vi "hex_tests.vi"() -> ()   [LabVIEW 2018]
panel:
  out "x > y?":bool
  out "concatenated string 3":string
  out "floor(x/y) 5":u32
  out "x-y*floor(x/y) 5":u32
  out "floor(x/y) 3":u32
  out "x-y*floor(x/y) 3":u32=2
  out "x-y*floor(x/y) 4":u32=12
  out "floor(x/y) 4":u32=18
  out "appended array 2":u32[](array[numeric])=[18, 12]
  out "string 3":string
  in  "y 2":u32=300
  in  "y":u32=300
  out "string 2":string
  out "appended array":u32[](array[numeric])=[1, 200]
  out "x+y":u32=200
  out "floor(x/y) 2":u32=1
  out "unsigned byte array":u8[](array[numeric])=[18, 12]
  out "string":string
  out "floor(x/y)":u32=18
  out "x-y*floor(x/y) 2":u32=2
  out "hex integer string":string="C"
  out "x-y*floor(x/y)":u32=12
  out "value":u32
  out "number":u32
  in  "hex":string="ý"
  out "offset past number 2":i32=1
  out "concatenated string":string
  out "number 3":u32=10
  out "decimal integer string":string="15"
  out "hex integer string 3":string="FFFFFFF1"
  out "hex integer string 2":string="F"
  out "offset past number":i32=1
  out "number 2":u32=9
  # "hex display makes out of 9 => 39"
  # "C"
  # "300 / 16 = 18,75 // 0,75 * 16 = 12"
  # "18 / 16 = 1,125 // 0,125 * 16 = 2"
  # "300 = 12C"
  # "4095 => FF0F wobei FF von unten"
  # "4096  => 0000 wobei unten überlauf bei IQ auf 16"
  # "4097 => 0001"
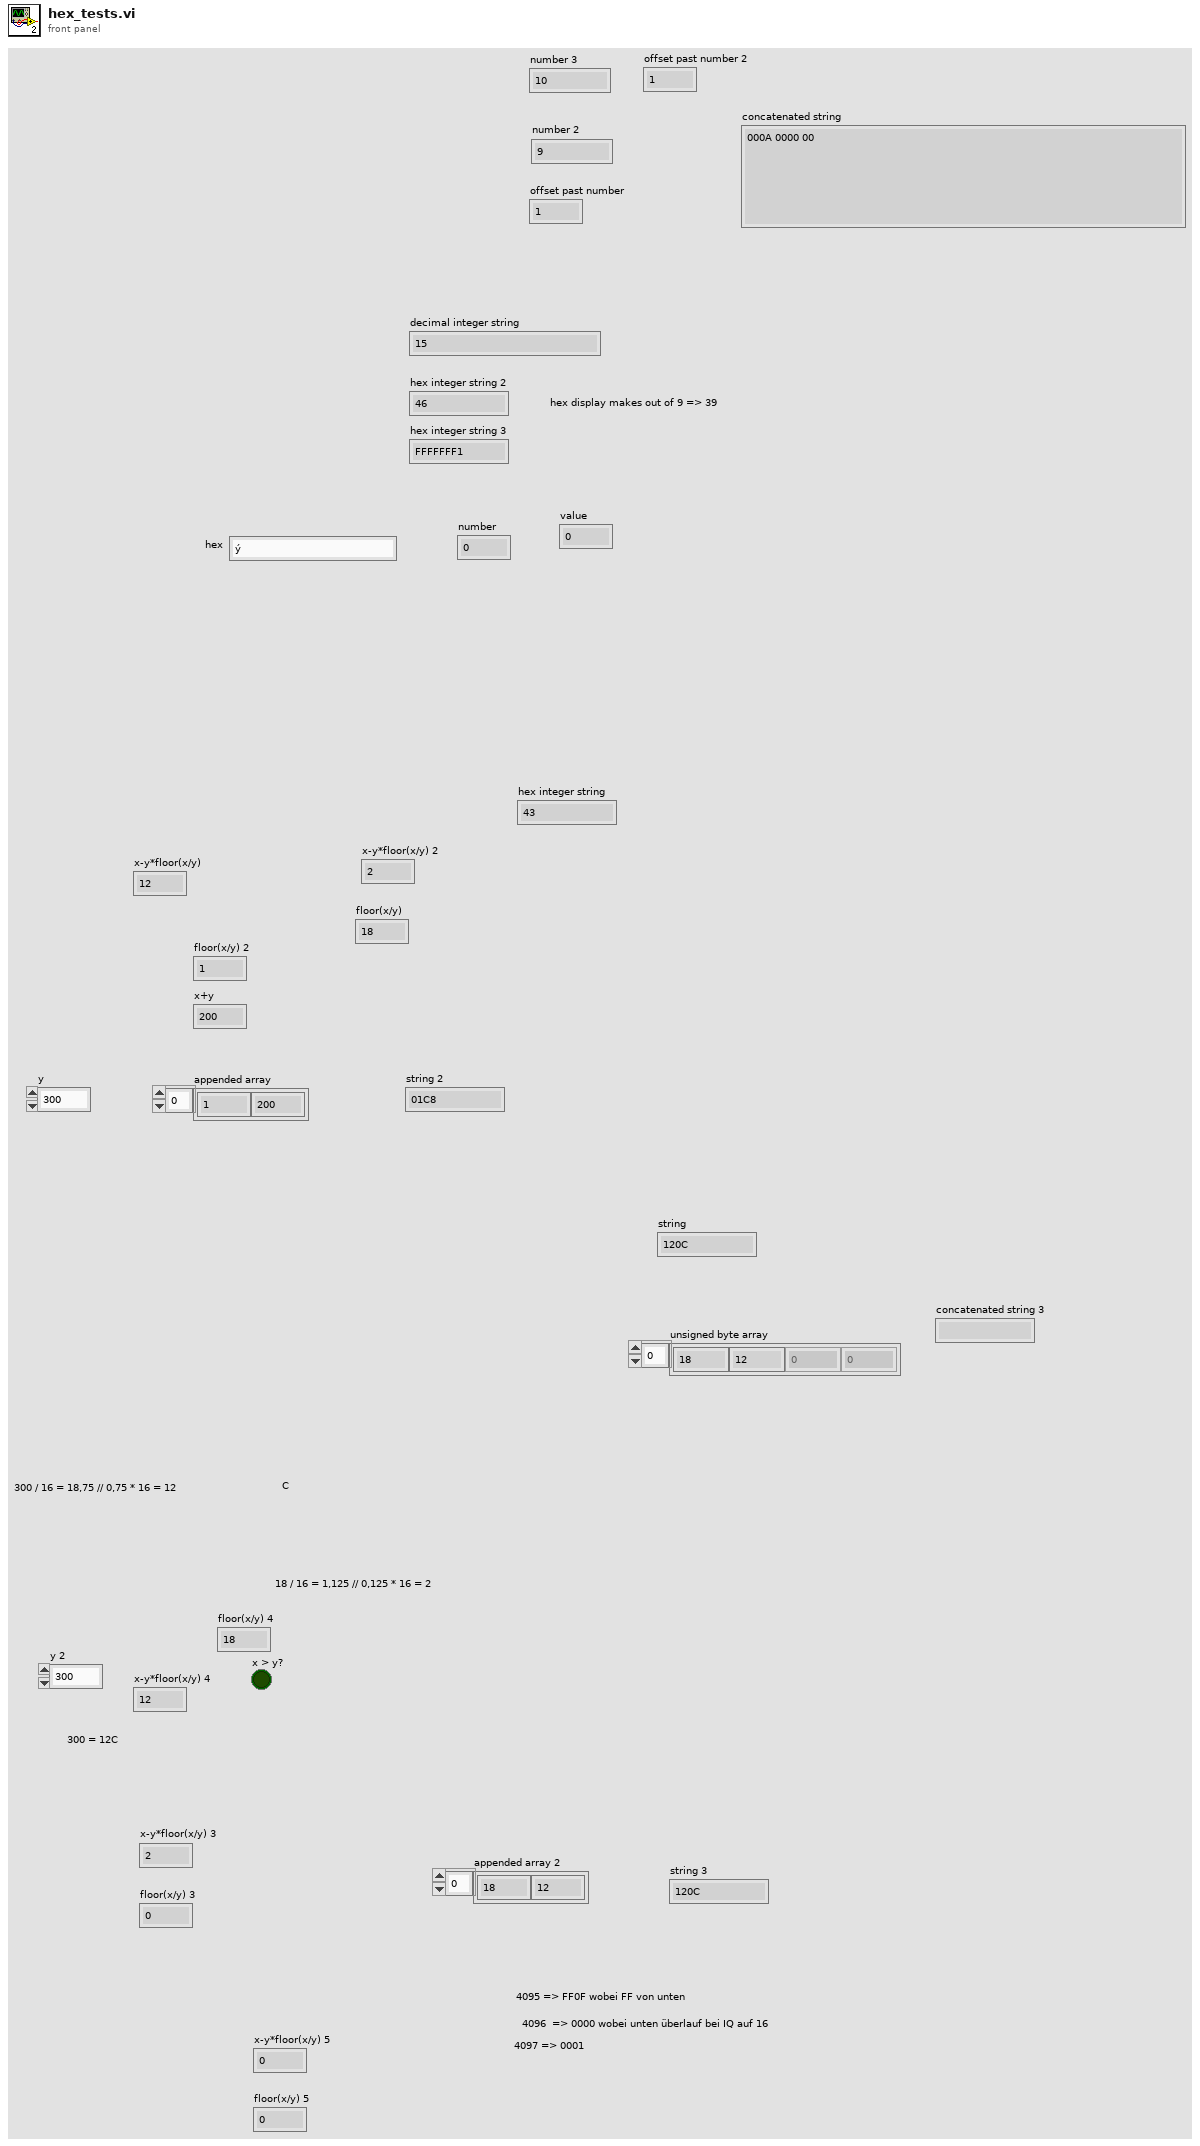
[diagram p1: front panel]
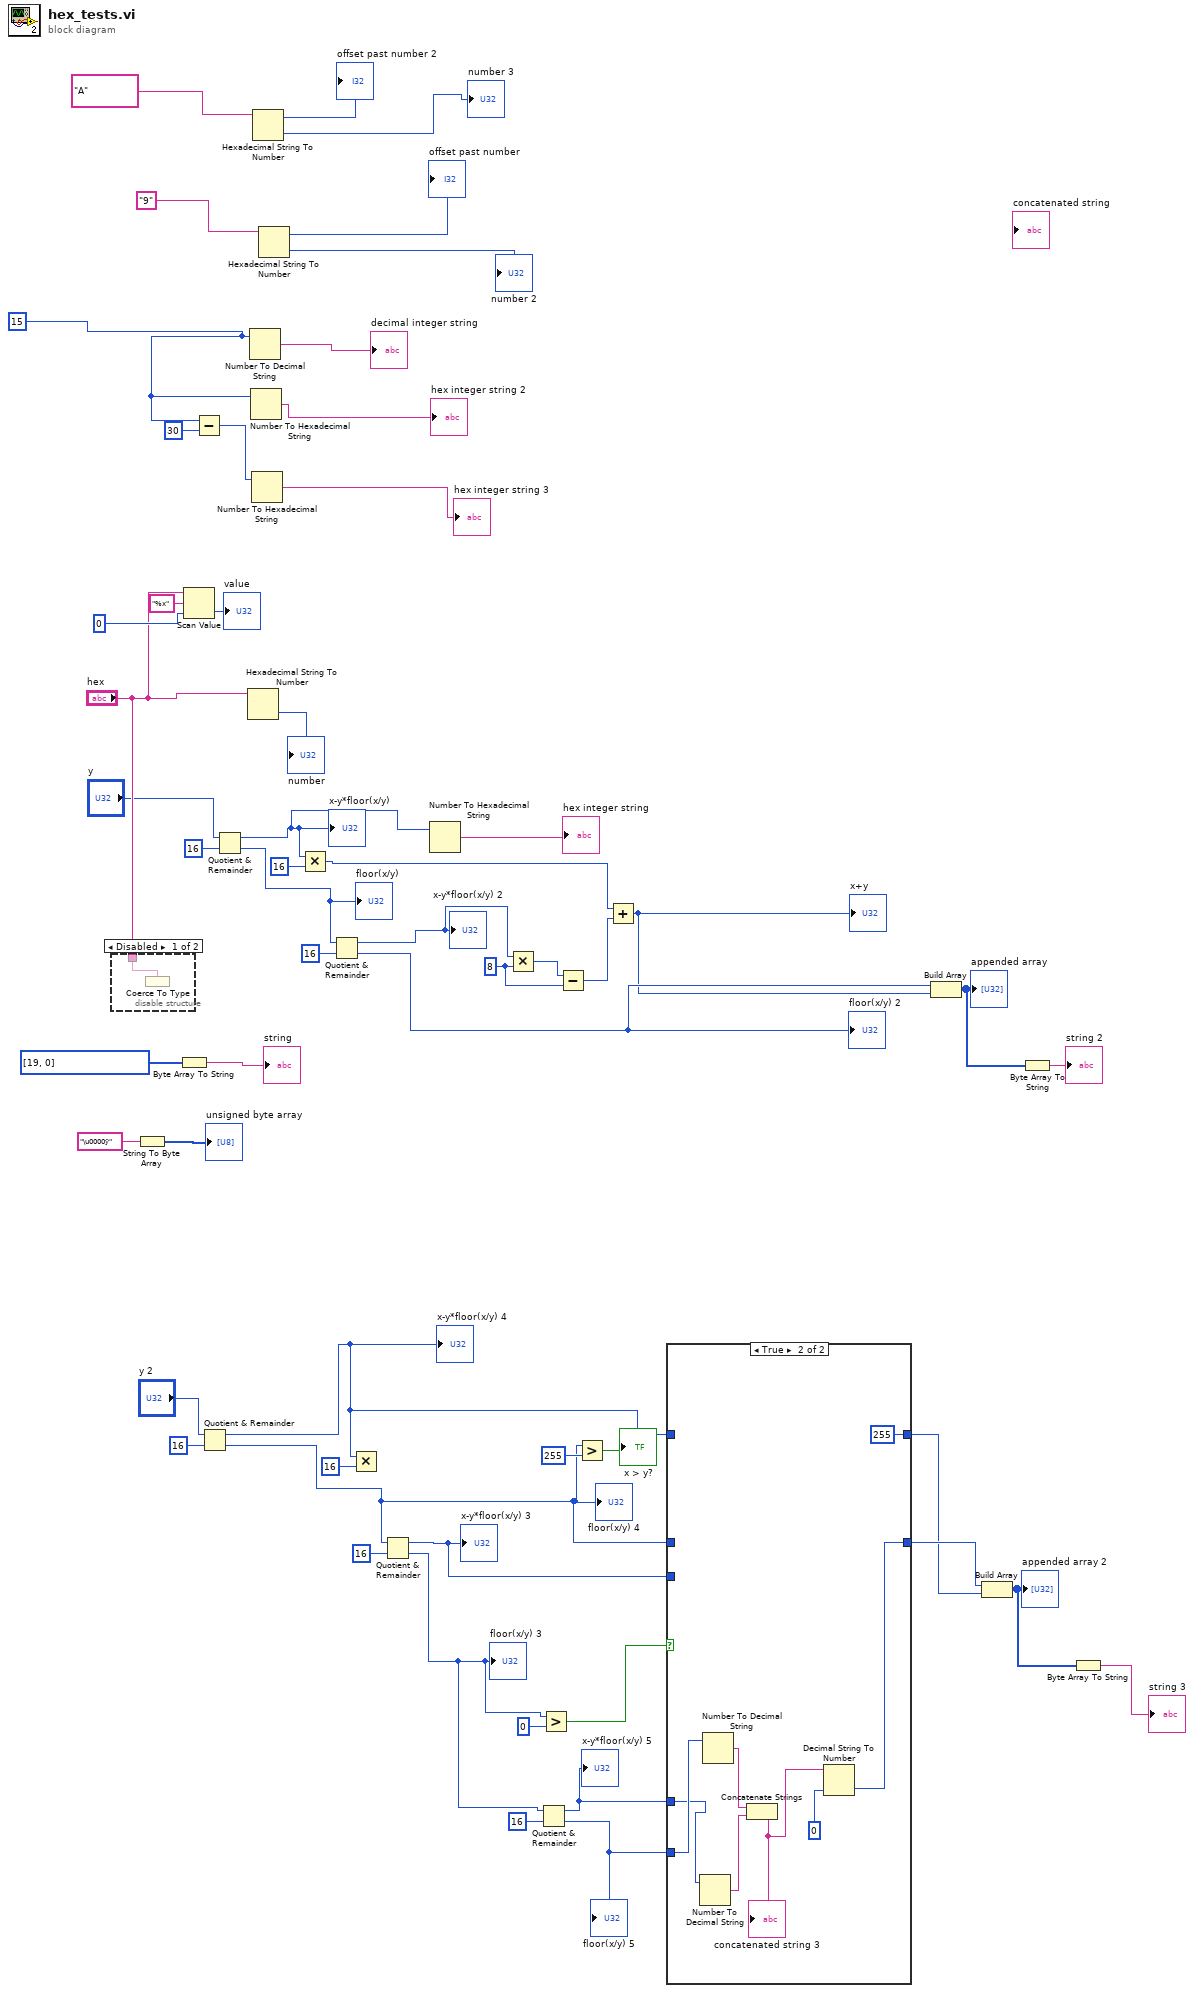
[diagram p0: block diagram]
diagram:
  w20 = u32 8 ("y")
  w45 = u32 15 ("number")
  n1 = disable-structure shown="Disabled" {
    disable-tunnel: "hex" -> [w57 _]
    frame Disabled {
      n2 = Coerce To Type(1:w57) -> ()  [unwired: 1 in, 1 out]
    }
    frame Enabled {
    }
  }
  n3 = String To Byte Array(string="\u0000ÿ") -> (unsigned byte array=→"unsigned byte array":u8[])
  n4 = Byte Array To String(unsigned byte array=u8[] [19, 0]) -> (string=→"string":string)
  n5 = Scan Value(string="hex", format string="%x", default (0 dbl)=u32 0 ("default (0 U32)")) -> (value=→"value":u32)  [unwired: 1 out]
  n6 = Subtract(x=w45, y=30) -> (x-y=w51:u32)
  n7 = Quotient & Remainder(x="y 2", y=u32 16) -> (x-y*floor(x/y)=w12:u32, floor(x/y)=w5:u32)
  "x-y*floor(x/y) 4" <- w12
  "floor(x/y) 4" <- w5
  n8 = Quotient & Remainder(x="y", y=u32 16) -> (x-y*floor(x/y)=w30:u32, floor(x/y)=w31:u32)
  "x-y*floor(x/y)" <- w30
  "floor(x/y)" <- w31
  n9 = Hexadecimal String To Number(string="hex") -> (number=→"number":u32)  [unwired: 2 in, 1 out]
  n10 = Number To Decimal String(number=w45) -> (decimal integer string=→"decimal integer string":string)  [unwired: 1 in]
  n11 = Number To Hexadecimal String(2:w45) -> (0:→"hex integer string 2":string)  [unwired: 1 in]
  n12 = Number To Hexadecimal String(2:w51) -> (0:→"hex integer string 3":string)  [unwired: 1 in]
  n13 = Hexadecimal String To Number(string="A" ("hex")) -> (offset past number=→"offset past number 2":i32, number=→"number 3":u32)  [unwired: 2 in]
  n14 = Hexadecimal String To Number(string="9" ("hex")) -> (offset past number=→"offset past number":i32, number=→"number 2":u32)  [unwired: 2 in]
  n15 = Multiply(x=w30, y=u32 16) -> (x*y=w27:u32)
  n16 = Quotient & Remainder(x=w31, y=u32 16) -> (x-y*floor(x/y)=w28:u32, floor(x/y)=w24:u32)
  "x-y*floor(x/y) 2" <- w28
  "floor(x/y) 2" <- w24
  n17 = Multiply(x=w12, y=u32 16) -> ()  [unwired: 1 out]
  n18 = Quotient & Remainder(x=w5, y=u32 16) -> (x-y*floor(x/y)=w10:u32, floor(x/y)=w2:u32)
  "x-y*floor(x/y) 3" <- w10
  "floor(x/y) 3" <- w2
  n19 = Number To Hexadecimal String(2:w30) -> (0:→"hex integer string":string)  [unwired: 1 in]
  n20 = Multiply(x=w28, y=w20) -> (x*y=w26:u32)
  n21 = Quotient & Remainder(x=w2, y=u32 16) -> (x-y*floor(x/y)=w7:u32, floor(x/y)=w8:u32)
  "x-y*floor(x/y) 5" <- w7
  "floor(x/y) 5" <- w8
  n22 = Greater?(x=w2, y=u32 0) -> (0:w1:bool)
  n23 = Subtract(x=w26, y=w20) -> (x-y=w25:u32)
  n24 = Greater?(x=w5, y=u32 255) -> (0:→"x > y?":bool)
  n25 = Add(x=w27, y=w25) -> (x+y=w23:u32)
  "x+y" <- w23
  n26 = case shown="True" w1 {
    tunnel: [w59 w61] -> w13
    tunnel: w5 -> [w59 _]
    tunnel: w12 -> [w58 _]
    tunnel: w10 -> [_ _]
    tunnel: w8 -> [_ w63]
    tunnel: w7 -> [_ w62]
    tunnel: [w58 u32 255] -> w6
    frame False {
    }
    frame True {
      n27 = Number To Decimal String(number=w62) -> (decimal integer string=w65:string)  [unwired: 1 in]
      n28 = Number To Decimal String(number=w63) -> (decimal integer string=w64:string)  [unwired: 1 in]
      n29 = Concatenate Strings(w64, w65) -> (w66:string)
      "concatenated string 3" <- w66
      n30 = Decimal String To Number(string=w66, default (0L)=u32 0 ("floor(x/y) 5")) -> (number=w61:u32)  [unwired: 1 in, 1 out]
    }
  }
  n31 = Build Array(w24, w23) -> (w22:u32[])
  "appended array" <- w22
  n32 = Build Array(w13, w6) -> (w18:u32[])
  "appended array 2" <- w18
  n33 = Byte Array To String(unsigned byte array=w22) -> (string=→"string 2":string)
  n34 = Byte Array To String(unsigned byte array=w18) -> (string=→"string 3":string)
